vi "ReadExEventWAIT.vi"() -> ()   [LabVIEW 2015]
uses:
  GPS_Driver_Global.vi
panel:
  in  "CloseWait":dbl
  in  "OpenWait":dbl
  in  "Path to FITS Header File":path=path "C:/Documents and Settings/observer/Desktop/timingtest.txt"
  out "# Entries After":i16
  in  "# Entries Before":i16
  out "Close Min":u32
  out "Close Maj":u32
  out "Open Min":u32
  out "Open Maj":u32
  out "error out":errorcluster
  in  "error in (no error)":errorcluster
  # "Major UNIX Time:"
  # "Minor UNIX Time:"
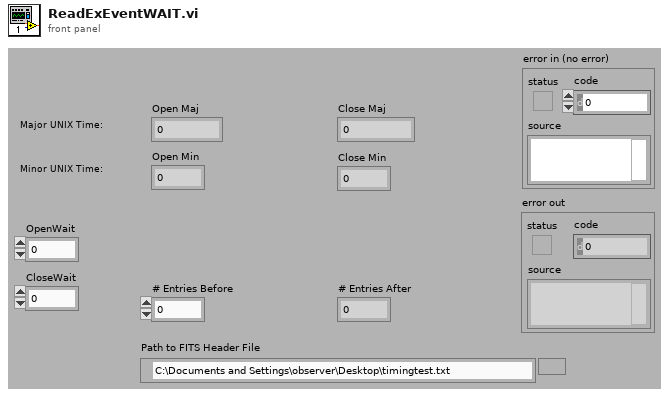
[diagram p1: front panel]
types:
  T1 = cluster{"Close":cluster{"Time":string, "Error":string}, "Open":cluster{"Time":string, "Error":string}}
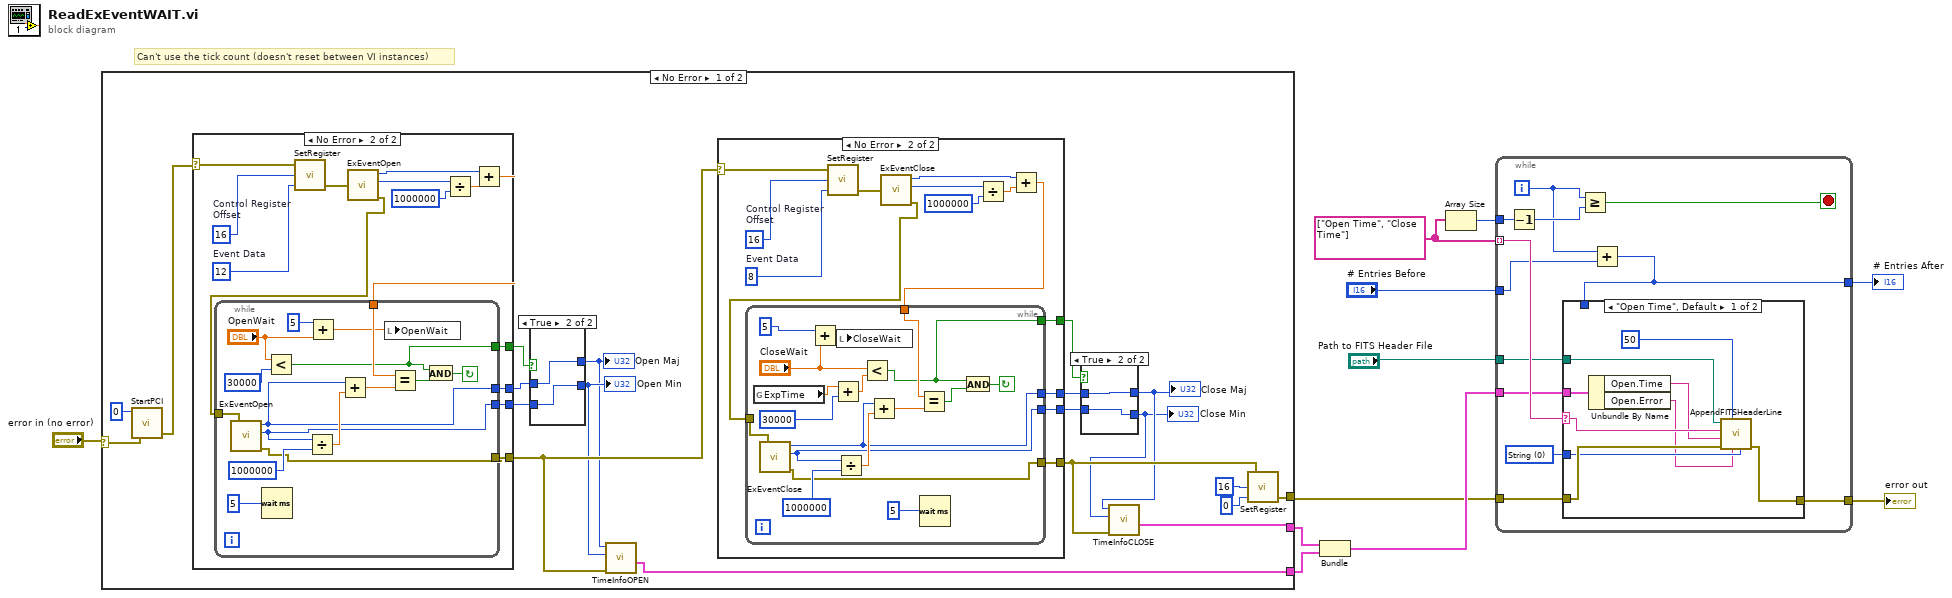
[diagram p0: block diagram]
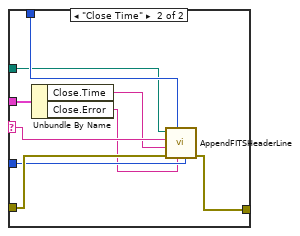
[diagram p2: hidden frame]
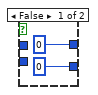
[diagram p3: hidden frame]
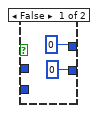
[diagram p4: hidden frame]
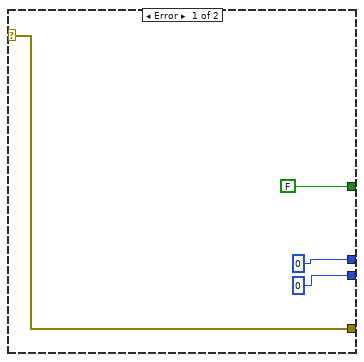
[diagram p5: hidden frame]
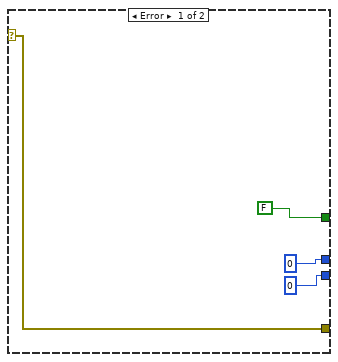
[diagram p6: hidden frame]
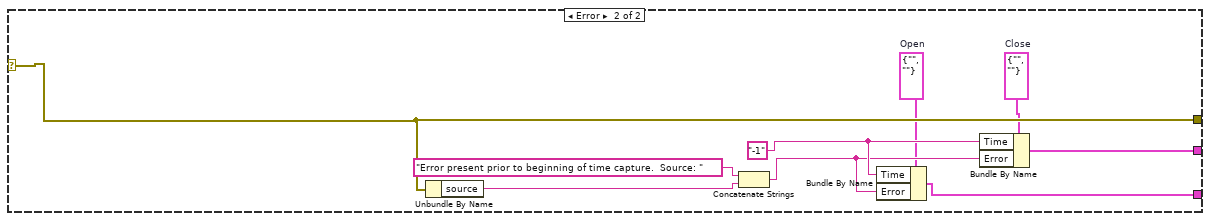
[diagram p7: hidden frame]
diagram:
  w11 = string[] ["Open Time", "Close Time"]
  # "Can't use the tick count (doesn't reset between VI instances)"
  n1 = case shown="No Error" "error in (no error)" {
    selector: "error in (no error)" -> [w22 w118]
    tunnel: [w28 w118] -> w6
    tunnel: [w27 w110] -> w7
    tunnel: [w25 w114] -> w8
    frame No Error {
      n2 = call "StartPCI.vi"("error in (no error)"=w22, "Device Number"=0) -> ("error out"=w24:errorcluster)  [unwired: 4 in]
      n3 = case shown="No Error" w24 {
        selector: w24 -> [w77 w81]
        tunnel: [0 w91] -> w18
        tunnel: [w77 w90] -> w23
        tunnel: [0 w89] -> w20
        tunnel: [FALSE w80] -> w21
        frame Error {
        }
        frame No Error {
          w92 = 12  # Event Data
          w93 = 16  # Control Register Offset
          n4 = call "SetRegister.vi"("Data"=w92, "Offset"=w93, "error in (no error)"=w81) -> ("error out"=w88:errorcluster)  [unwired: 2 in]
          n5 = call "ExEventOpen.vi"("error in (no error)"=w88) -> ("Major Time"=w84:u32, "Minor Time"=w87:u32, "error out"=w85:errorcluster)  [unwired: 1 in]
          n6 = Divide(x=w87, y=1000000) -> (x/y=w83:dbl)
          n7 = Add(x=w84, y=w83) -> (x+y=w82:dbl)
          n8 = while {
            tunnel: w85 -> [w109]
            tunnel: w82 -> [w108]
            tunnel: [w105] -> w90
            tunnel: [w95] -> w89
            tunnel: [w94] -> w91
            tunnel: [w96] -> w80
            stop <- w102 continue-if-true
            n9 = call "ExEventOpen.vi"("error in (no error)"=w109) -> ("Major Time"=w95:u32, "Minor Time"=w94:u32, "error out"=w105:errorcluster)  [unwired: 1 in]
            n10 = Wait (ms)(milliseconds to wait=5) -> ()  [unwired: 1 out]
            n11 = Less?(x="OpenWait", y=30000) -> (x < y?=w96:bool)
            n12 = Divide(x=w94, y=1000000) -> (x/y=w107:dbl)
            n13 = Add(x=5, y="OpenWait") -> (x+y=w97:dbl)
            n14 = Add(x=w95, y=w107) -> (x+y=w104:dbl)
            n15 = local write "OpenWait"(w97) -> ()
            n16 = Equal?(x=w108, y=w104) -> (x = y?=w101:bool)
            n17 = And(x=w96, y=w101) -> (x .and. y?=w102:bool)
          }
        }
      }
      n18 = case shown="True" w21 {
        tunnel: w20 -> [_ w38]
        tunnel: [0 w39] -> w19
        tunnel: w18 -> [_ w39]
        tunnel: [0 w38] -> w17
        frame False {
        }
        frame True {
        }
      }
      "Open Min" <- w19
      "Open Maj" <- w17
      n19 = call "TimeInfoOPEN.vi"("error in (no error)"=w23, "Minor Time"=w19, "Major Time"=w17) -> ("Open"=w27:cluster{"Time":string, "Error":string})  [unwired: 6 in, 1 out]
      n20 = case shown="No Error" w23 {
        selector: w23 -> [w41 w45]
        tunnel: [0 w55] -> w12
        tunnel: [w41 w54] -> w26
        tunnel: [0 w53] -> w14
        tunnel: [FALSE w44] -> w16
        frame Error {
        }
        frame No Error {
          w56 = 8  # Event Data
          w57 = 16  # Control Register Offset
          n21 = call "SetRegister.vi"("Data"=w56, "Offset"=w57, "error in (no error)"=w45) -> ("error out"=w52:errorcluster)  [unwired: 2 in]
          n22 = call "ExEventClose.vi"("error in (no error)"=w52) -> ("Major Time"=w48:u32, "Minor Time"=w51:u32, "error out"=w49:errorcluster)  [unwired: 1 in]
          n23 = Divide(x=w51, y=1000000) -> (x/y=w47:dbl)
          n24 = Add(x=w48, y=w47) -> (x+y=w46:dbl)
          n25 = while {
            tunnel: w49 -> [w75]
            tunnel: w46 -> [w74]
            tunnel: [w71] -> w54
            tunnel: [w68] -> w53
            tunnel: [w70] -> w55
            tunnel: [w58] -> w44
            stop <- w63 continue-if-true
            n26 = global read "GPS_Driver_Global.vi" "ExpTime"() -> (w67:dbl)
            n27 = call "ExEventClose.vi"("error in (no error)"=w75) -> ("Major Time"=w68:u32, "Minor Time"=w70:u32, "error out"=w71:errorcluster)  [unwired: 1 in]
            n28 = Add(x=5, y="CloseWait") -> (x+y=w59:dbl)
            n29 = Add(x=w67, y=30000) -> (x+y=w65:dbl)
            n30 = Divide(x=w70, y=1000000) -> (x/y=w73:dbl)
            n31 = local write "CloseWait"(w59) -> ()
            n32 = Less?(x="CloseWait", y=w65) -> (x < y?=w58:bool)
            n33 = Add(x=w68, y=w73) -> (x+y=w69:dbl)
            n34 = Equal?(x=w74, y=w69) -> (x = y?=w64:bool)
            n35 = Wait (ms)(milliseconds to wait=5) -> ()  [unwired: 1 out]
            n36 = And(x=w58, y=w64) -> (x .and. y?=w63:bool)
          }
        }
      }
      n37 = case shown="True" w16 {
        tunnel: [0 w35] -> w15
        tunnel: w14 -> [_ w35]
        tunnel: [0 w34] -> w13
        tunnel: w12 -> [_ w34]
        frame False {
        }
        frame True {
        }
      }
      "Close Maj" <- w15
      "Close Min" <- w13
      n38 = call "TimeInfoCLOSE.vi"("error in (no error)"=w26, "Minor Time"=w13, "Major Time"=w15) -> ("Close"=w25:cluster{"Time":string, "Error":string})  [unwired: 7 in]
      n39 = call "SetRegister.vi"("Data"=0, "Offset"=16, "error in (no error)"=w26) -> ("error out"=w28:errorcluster)  [unwired: 2 in]
    }
    frame Error {
      w115 = cluster{"Time":string, "Error":string} {"Time"="", "Error"=""}  # Close
      w111 = cluster{"Time":string, "Error":string} {"Time"="", "Error"=""}  # Open
      w113 = "-1"
      n40 = Unbundle By Name(w118) -> ("source"=w116:string)
      n41 = Concatenate Strings("Error present prior to beginning of time capture.  Source: ", w116) -> (w112:string)
      n42 = Bundle By Name(cluster=w111, "Time"=w113, "Error"=w112) -> (w110:cluster{"Time":string, "Error":string})
      n43 = Bundle By Name(cluster=w115, "Time"=w113, "Error"=w112) -> (w114:cluster{"Time":string, "Error":string})
    }
  }
  n44 = Bundle("Close"=w8, "Open"=w7) -> (w10:T1)  [unwired: 1 in]
  n45 = Array Size(array=w11) -> (size(s)=w4:i32)
  n46 = while {
    tunnel: w6 -> [w130]
    tunnel: w11 -> [w128] mode=indexing
    tunnel: w4 -> [w127]
    tunnel: "# Entries Before" -> [w125]
    tunnel: w10 -> [w123]
    tunnel: "Path to FITS Header File" -> [w122]
    tunnel: [w121] -> w9
    tunnel: [w120] -> w2
    i -> [w124]
    stop <- w119 stop-if-true
    w126 = u16 0 items=["String", "Numeric", "Boolean"]
    n47 = Decrement(x=w127) -> (x-1=w129:i32)
    n48 = Greater Or Equal?(x=w124, y=w129) -> (x >= y?=w119:bool)
    n49 = Add(x=w124, y=w125) -> (x+y=w120:i32)
    n50 = case shown="\"Open Time\", Default" w128 {
      selector: w128 -> [w137 w147]
      tunnel: w130 -> [w139 w148]
      tunnel: w126 -> [w138 w146]
      tunnel: w123 -> [w134 w142]
      tunnel: w120 -> [_ w144]
      tunnel: w122 -> [w136 w143]
      tunnel: [w135 w145] -> w121
      frame "Open Time", Default {
        n51 = Unbundle By Name(w134) -> ("Open.Time"=w133:string, "Open.Error"=w132:string)
        n52 = call "AppendFITSHeaderLine.vi"("Entry Type"=w138, "Comment"=w132, "Entry #"=50, "error in (no error)"=w139, "Element Value"=w133, "Element Name"=w137, "file path (dialog if empty)"=w136) -> ("error out"=w135:errorcluster)  [unwired: 3 in]
      }
      frame "Close Time" {
        n53 = Unbundle By Name(w142) -> ("Close.Time"=w141:string, "Close.Error"=w140:string)
        n54 = call "AppendFITSHeaderLine.vi"("Entry Type"=w146, "Comment"=w140, "Entry #"=w144, "error in (no error)"=w148, "Element Value"=w141, "Element Name"=w147, "file path (dialog if empty)"=w143) -> ("error out"=w145:errorcluster)  [unwired: 3 in]
      }
    }
  }
  "error out" <- w9
  "# Entries After" <- w2
